vi "Open.vi"(8 "error in (no error)":errorcluster, 11 "Server in":refnum<class "Server.lvclass">) -> (0 "error out":errorcluster, 3 "Server out":refnum<class "Server.lvclass">)   [LabVIEW 2020, in "HTTP Server.lvlib" / "Server.lvclass"]
uses:
  Server.lvclass
  Server.lvclass/Server.ctl
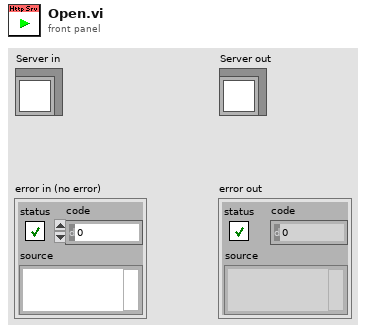
[diagram p1: front panel]
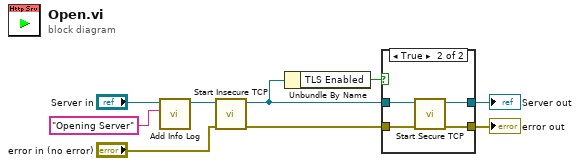
[diagram p0: block diagram]
diagram:
  n1 = call "Add Info Log.vi"("Info"="Opening Server", "Server in"="Server in") -> ("Server out"=w8:refnum<class "Server.lvclass">)  [unwired: 8 in, 1 out]
  n2 = call "Start Insecure TCP.vi"("error in (no error)"="error in (no error)", "Server in"=w8) -> ("error out"=w2:errorcluster, "Server out"=w6:refnum<class "Server.lvclass">)  [unwired: 8 in]
  n3 = Unbundle By Name(w6) -> ("TLS Enabled"=w3:bool)
  n4 = case shown="True" w3 {
    tunnel: w6 -> [w11 w15]
    tunnel: [w11 w14] -> w4
    tunnel: w2 -> [w10 w13]
    tunnel: [w10 w12] -> w1
    frame False {
    }
    frame True {
      n5 = call "Start Secure TCP.vi"("error in (no error)"=w13, "Server in"=w15) -> ("error out"=w12:errorcluster, "Server out"=w14:refnum<class "Server.lvclass">)  [unwired: 8 in]
    }
  }
  "error out" <- w1
  "Server out" <- w4
